vi "ASAP.vi"() -> ()   [LabVIEW 2011]
doc: "I. Description:\nThis example demonstrates how to acquire a continuous amount of data (Waveform) using the DAQ device's internal clock.\n\nII. Instructions for Running:\n1. Create an analog input voltage channel.\n2. Set the rate for the sample clock. Additionally, define the sample mode to be continuous.\n3. Call the Start VI to start the acquisition.\n4. Read the waveform data in a loop until the user hits the stop button or an error occurs.\nNote: This example reads data from one or more channels and returns an array of data. Use the Index Array function to access an individual channel of data.\n5. Call the Clear Task VI to clear the Task.\n6. Use the popup dialog box to display an error if any.\n\nIV. I/O Connections Overview:\nMake sure your signal input terminal matches the Physical Channel I/O Control. For further connection information, refer to your hardware reference manual."
uses:
  micron/labview/manipulator/squiggle/Host/fpga_reference.ctl
  micron/labview/manipulator/squiggle/Host/i2c_interface.ctl
  micron/labview/cancellation/estimation_controls.ctl
  micron/labview/cancellation/sq_control_params.ctl
  micron/labview/filtering/goal_loop_parms.ctl
  micron/labview/host/network_params.ctl
  probe_calibration.ctl
  micron/labview/testing/manipulator_cal.ctl
  micron/labview/testing/mode_conrols.ctl
  micron/labview/testing/injection_point.ctl
  micron/labview/testing/stimulus.ctl
  micron/labview/testing/Micron params.ctl
  micron/labview/initialization/micron_config.ctl
  initialization/globals.vi
panel:
  in  "Use LUT":bool
  in  "Finder":bool
  in  "Microns full scale":dbl=12000.0
  in  "Light enables":bool[](array[boolean])=[TRUE, TRUE, FALSE, FALSE]
  out "Logging":bool
  in  "3D Curve":refnum<k7>(container)
  in  "Offset mode":enum32{"Absolute", "Relative"}(radio)
  in  "Zero":bool
  out "Position":cluster{"X":dbl, "Y":dbl, "Z":dbl} {"Z" format="%#5.0f"; "Y" format="%#5.0f"; "X" format="%#5.0f"}
  out "Angles":cluster{"Altitude":dbl, "Azimuth":dbl} {"Azimuth" format="%7.2f"; "Altitude" format="%7.2f"}
  in  "Ref point offset":dbl
  in  "Point selection":enum16{"Light 0", "Light 1", "Ref point"}(ring)
  out "Status":cluster{"Valid position":bool, "Message":string}
  in  "Stop Logging":bool
  in  "Continuous Log":bool
  in  "Start Timed Log":bool
  in  "Log duration":dbl
  in  "Log File":path
  out "XYZ offsets":waveform(dbl)[](graph)
  in  "stop":bool
  # "(degrees)"
  # "(microns)"
  # "Logging"
  # "Log duration (sec):"
  # "(mm)"
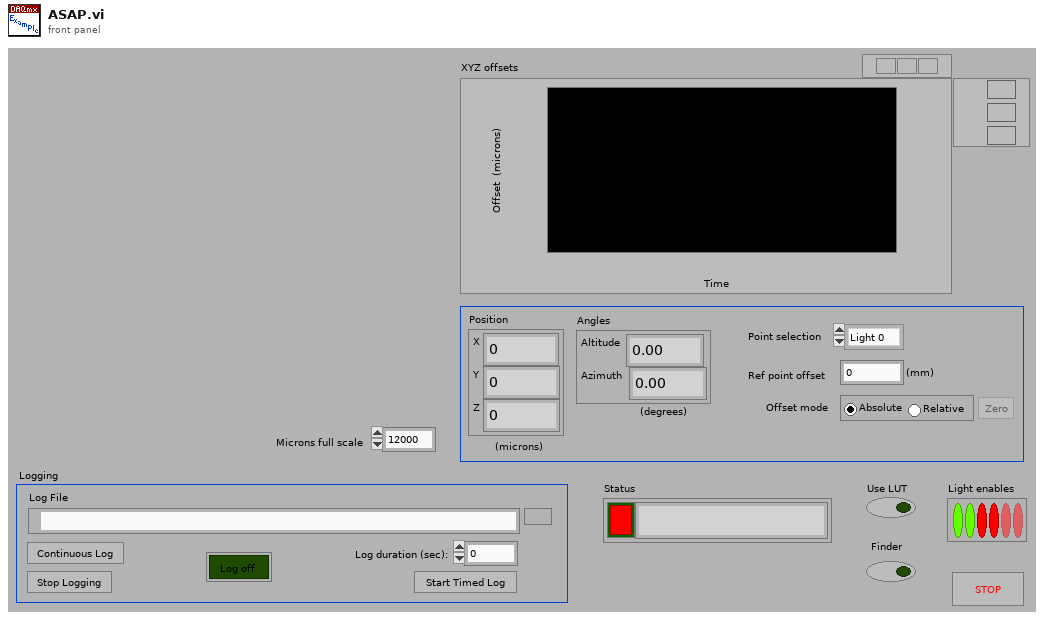
[diagram p1: front panel]
types:
  T1 = enum16{"ASAP/Trigger", "ASAP/Finder", "ASAP/Micron", "ASAP/Micron 2", "Micron 6DOF"}
  T2 = typedef "configuration.ctl" = cluster{"Calibration data":cluster{"T1":T3, "K1":T3, "T2":T3, "K2":T3}, "Block size":i32, "Tasks":cluster{"Analog Input":refnum<k21>, "Counters":refnum<k21>[], "Digital out":refnum<k21>}, "Light enables":bool[], "Demodulator table":dbl[][][]}
  T3 = typedef "NI_Matrix.lvlib/RealMatrix.ctl" = dbl[][]
  T4 = typedef "i2c_interface.ctl" = cluster{"FPGA VI Reference":T5}
  T5 = typedef "fpga_reference.ctl" = refnum<k20>
  T6 = typedef "micron_config.ctl" = cluster{"rt fifo":refnum<k33>, "Analog output task":refnum<k21>, "Analog output task 2":refnum<k21>, "Stimulus AO task":refnum<k21>, "Low-rate AIN task":refnum<k21>, "Pedal out task":refnum<k21>, "Pedal in task":refnum<k21>, "Loop timing source":string, "Relay out task":refnum<k21>, "Send UDP Conn":refnum<k16>, "Recv UDP Conn":refnum<k16>, "Host Addr":dbl, "I2C interface":T4, "trace_start notifier":refnum<notifier>, "trace_done notifier":refnum<notifier>, "ASAP FIFO":refnum<k33>}
  T7 = cluster{"Analog Input":refnum<k21>, "Counters":refnum<k21>[], "Digital out":refnum<k21>}
  T8 = cluster{"X values":waveform(dbl), "Y values":waveform(dbl), "Z values":waveform(dbl)}[]
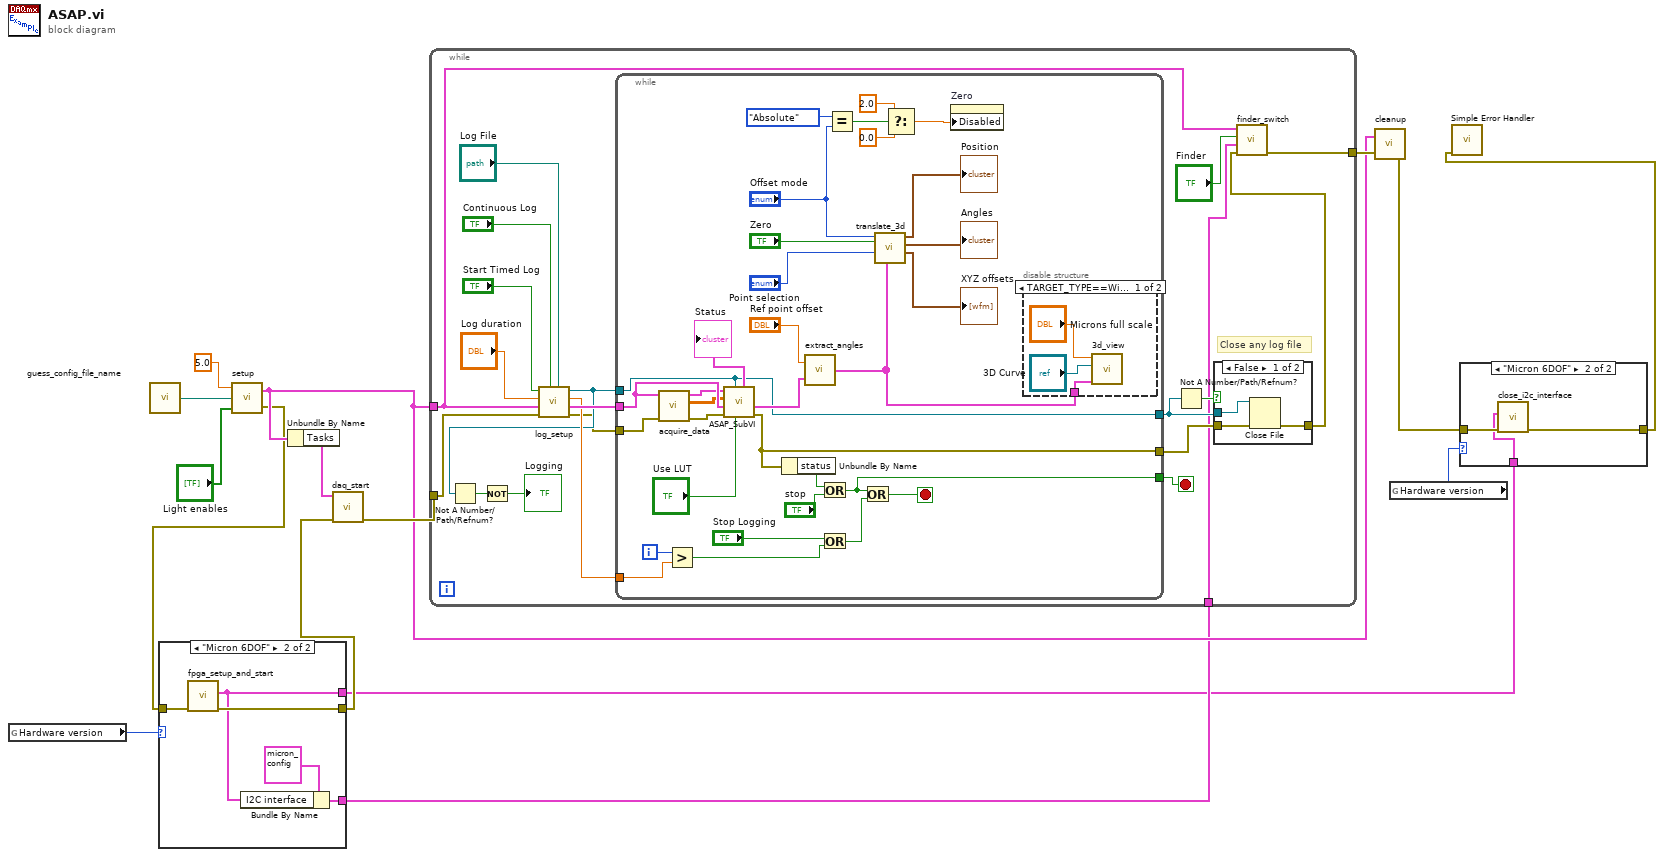
[diagram p0: block diagram]
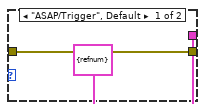
[diagram p3: hidden frame]
diagram:
  n1 = global read "globals.vi" "Hardware version"() -> (w8:T1)
  n2 = call "guess_config_file_name.vi"() -> ("config file path"=w12:path)
  n3 = call "setup.vi"("Light enables"="Light enables", "Calibration file name"=w12, "Updates/sec"=5.0) -> ("error out"=w7:errorcluster, "Configuration"=w9:T2)  [unwired: 1 out]
  n4 = case shown="\"Micron 6DOF\"" w8 {
    tunnel: w7 -> [w17 w22]
    tunnel: [w17 w21] -> w6
    tunnel: [T4 {"FPGA VI Reference"=refnum} ("I2C interface") w19] -> w1
    tunnel: [_ w18] -> w2
    frame "ASAP/Trigger", Default {
    }
    frame "Micron 6DOF" {
      n5 = call "fpga_setup_and_start.vi"("error in"=w22) -> ("error out"=w21:errorcluster, "I2C interface"=w19:T4)  [unwired: 9 in]
      n6 = Bundle By Name(cluster=T6 {"rt fifo"=refnum, "Analog output task"="", "Analog output task 2"="", "Stimulus AO task"="", "Low-rate AIN task"="", "Pedal out task"="", "Pedal in task"="", "Loop timing source"="", "Relay out task"="", "Send UDP Conn"=refnum, "Recv UDP Conn"=refnum, "Host Addr"=0.0, "I2C interface"={"FPGA VI Reference"=refnum}, "trace_start notifier"=refnum, "trace_done notifier"=refnum, "ASAP FIFO"=refnum} ("Micron config"), "I2C interface"=w19) -> (w18:T6)
    }
  }
  n7 = Unbundle By Name(w9) -> ("Tasks"=w11:T7)
  n8 = call "daq_start.vi"("error in"=w6, "Tasks"=w11) -> ("error out"=w10:errorcluster)  [unwired: 9 out]
  n9 = while {
    tunnel: w9 -> [w27]
    tunnel: [w24] -> w15
    tunnel: w10 -> [w28]
    tunnel: w2 -> [w23]
    stop <- w42 stop-if-true
    # "Close any log file"
    n10 = call "log_setup.vi"("Log File"="Log File", "Continuous Log"="Continuous Log", "error in"=w28, "Configuration"=w27, "Log duration"="Log duration", "Start Timed Log"="Start Timed Log") -> ("error out"=w29:errorcluster, "Configuration Out"=w32:T2, "Loop count"=w31:dbl, "refnum out"=w30:refnum<file>)  [unwired: 1 in, 1 out]
    n11 = Not A Number/Path/Refnum?(number/path/refnum=w30) -> (NaN/Path/Refnum?=w38:bool)
    n12 = Not(x=w38) -> (.not. x?=→"Logging":bool)
    n13 = while {
      tunnel: w32 -> [w50]
      tunnel: [w77] -> w41
      tunnel: [w75] -> w42
      tunnel: w30 -> [w51]
      tunnel: w31 -> [w69]
      tunnel: [w51] -> w39
      tunnel: w29 -> [w52]
      i -> [w70]
      stop <- w74 stop-if-true
      n14 = call "acquire_data.vi"("error in"=w52, "Configuration"=w50) -> ("error out"=w53:errorcluster, "Data"=w48:dbl[][], "timestamp"=w49:cluster{"t0":timestamp, "dt":dbl})  [unwired: 5 out]
      n15 = Greater?(x=w70, y=w69) -> (0:w72:bool)
      n16 = call "ASAP_SubVI.vi"("Use LUT"="Use LUT", "Log file refnum"=w51, "error in"=w53, "Configuration"=w50, "ADC data"=w48, "timestamp"=w49) -> ("error out"=w77:errorcluster, "XYZ out"=w56:T8, "Diagnostics"=→"Status":cluster{"Valid position":bool, "Message":string})  [unwired: 3 out]
      n17 = Unbundle By Name(w77) -> ("status"=w76:bool)
      n18 = call "extract_angles.vi"("Ref point offset (mm)"="Ref point offset", "XYZ in, two points"=w56) -> ("points out"=w54:T8)  [unwired: 2 out]
      n19 = Or(x=w76, y="stop") -> (x .or. y?=w75:bool)
      n20 = Or(x="Stop Logging", y=w72) -> (x .or. y?=w71:bool)
      n21 = Equal?(x=enum32{"Absolute", "Relative"}."Absolute", y="Offset mode") -> (x = y?=w61:bool)
      n22 = Or(x=w75, y=w71) -> (x .or. y?=w74:bool)
      n23 = call "translate_3d.vi"("XYZ position"=w54, "Point selection"="Point selection", "Zero"="Zero", "Offset mode"="Offset mode") -> ("XYZ offsets"=→"XYZ offsets":waveform(dbl)[], "Angles"=→"Angles":cluster{"Altitude":dbl, "Azimuth":dbl}, "Position"=→"Position":cluster{"X":dbl, "Y":dbl, "Z":dbl})  [unwired: 5 out]
      n24 = Select(t=2.0, s=w61, f=0.0) -> (s? t:f=w60:dbl)
      n25 = property on="Zero" class="Bool"("Disabled"=w60) -> ()  [unwired: 2 in, 2 out]
      n26 = disable-structure shown="TARGET_TYPE==Windows" {
        disable-tunnel: w54 -> [w80 _]
        frame condition #0 (active) {
          n27 = call "3d_view.vi"("3D values"=w80, "3D Curve"="3D Curve", "3D view scale"="Microns full scale") -> ()  [unwired: 3 out]
        }
        frame condition #1 {
        }
      }
    }
    n28 = Not A Number/Path/Refnum?(number/path/refnum=w39) -> (NaN/Path/Refnum?=w40:bool)
    n29 = case shown="False" w40 {
      tunnel: w41 -> [w45 w46]
      tunnel: [w44 w46] -> w25
      tunnel: w39 -> [w43 _]
      frame False {
        n30 = Close File(refnum=w43, error in=w45) -> (error out=w44:errorcluster)  [unwired: 1 out]
      }
      frame True {
      }
    }
    n31 = call "finder_switch.vi"("error in"=w25, "Micron config"=w23, "Finder"="Finder", "Configuration"=w27) -> ("error out"=w24:errorcluster)  [unwired: 5 out]
  }
  n32 = call "cleanup.vi"("error in"=w15, "Configuration"=w9) -> ("error out"=w4:errorcluster)  [unwired: 1 out]
  n33 = global read "globals.vi" "Hardware version"() -> (w5:T1)
  n34 = case shown="\"Micron 6DOF\"" w5 {
    tunnel: [w82 w85] -> w3
    tunnel: w4 -> [w82 w84]
    tunnel: w1 -> [_ w83]
    frame "ASAP/Trigger", Default {
    }
    frame "Micron 6DOF" {
      n35 = call "close_i2c_interface.vi"("error in"=w84, "I2C interface"=w83) -> ("error out"=w85:errorcluster)  [unwired: 9 in]
    }
  }
  n36 = call <vilib>:"Simple Error Handler.vi"("error in (no error)"=w3) -> ()  [unwired: 1 in, 8 out]
